vi "Webcam Management.vi"() -> ()   [LabVIEW 2014]
uses:
  <vilib>/vision/driver/IMAQdx.llb/IMAQdx Attribute Type.ctl
  <vilib>/userdefined/High Color/IMAQdx.ctl
  <vilib>/vision/driver/NI_Vision_Acquisition_Software.lvlib
  <resource>/objmgr/imaqdx.rc
panel:
  out "Brightness Mode":u32
  out "Contrast Mode":u32
  in  "Brightness":dbl
  in  "Contrast":dbl min=0.0 max=0.6 step=0.1
  out "Attribute Information Array":T2(array[cluster])
  out "Image":T3(plugin-control)
  in  "stop":bool
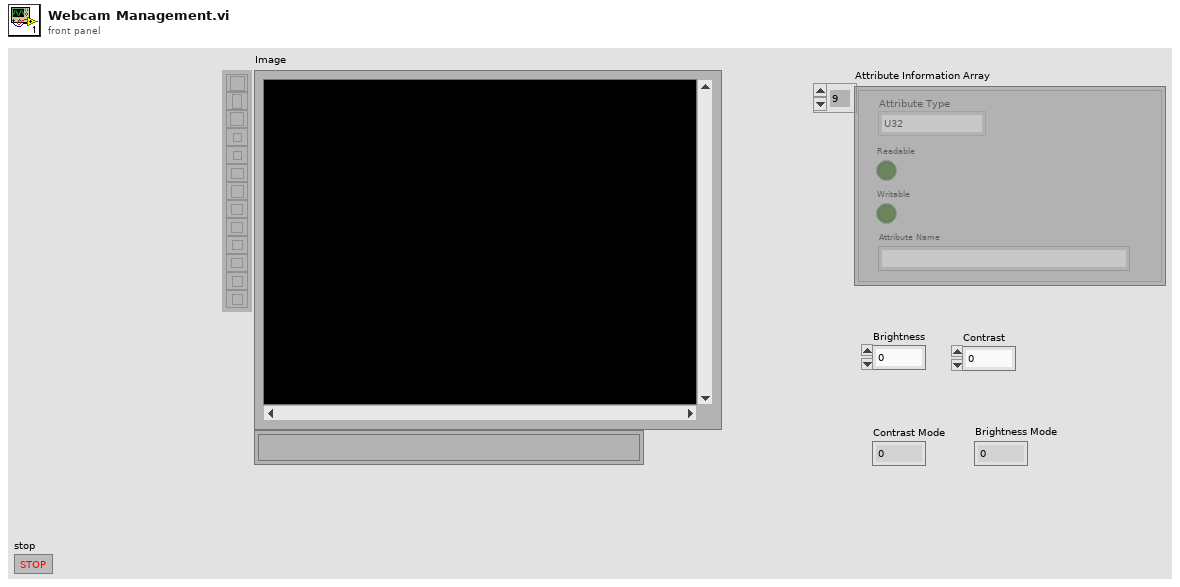
[diagram p1: front panel]
types:
  T1 = typedef "NI_Vision_Acquisition_Software.lvlib/IMAQdx Attribute Type.ctl" = enum32{"U32", "I64", "DBL", "String", "Enum", "Bool", "Command"}
  T2 = cluster{"Attribute Type":T1, "Readable":bool, "Writable":bool, "Attribute Name":string}[]
  T3 = typedef "IMAQ Image.ctl" = refnum<image>
  T4 = typedef "Image Type" = u32
  T5 = typedef "IMAQdx.ctl" = refnum<k21>
  T6 = cluster{"Global Rectangle":i32[], "Contours":cluster{"Contour Type":u32, "ROI Type":u32, "Points":i32[]}[]}
  T7 = cluster{"Global Rectangle[0]":i32, "Global Rectangle[1]":i32, "Global Rectangle[2]":i32, "Global Rectangle[3]":i32}
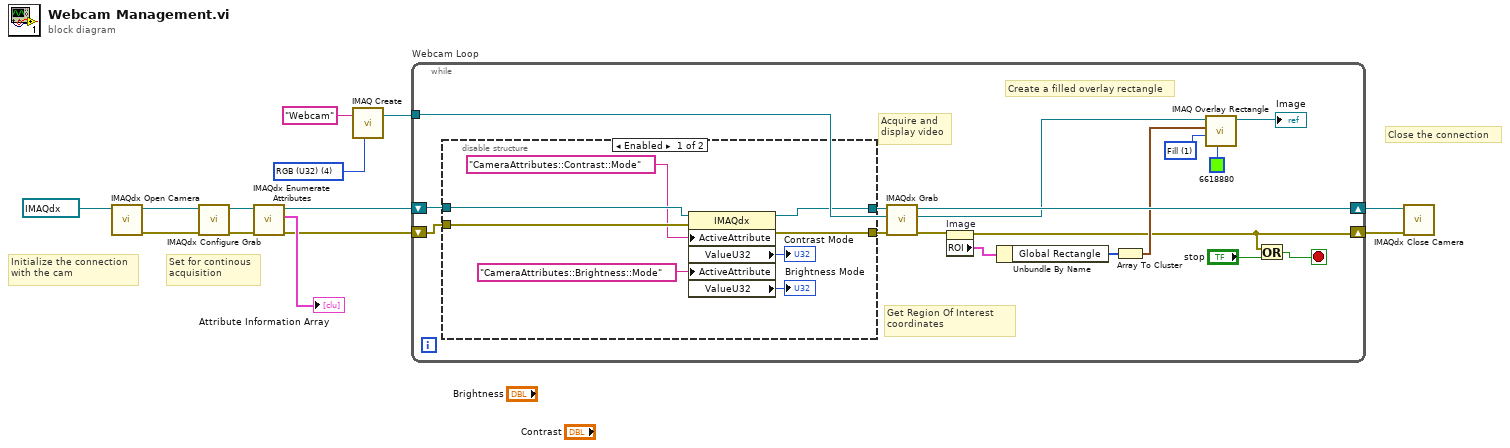
[diagram p0: block diagram]
diagram:
  w7 = T4 4 items=["Grayscale (U8)", "Grayscale (I16)", "Grayscale (SGL)", "Complex (CSG)", "RGB (U32)", "HSL (U32)", "RGB (U64)", "Grayscale (U16)"] ("Image Type")
  # "Close the connection"
  # "Set for continous\nacquisition"
  # "Initialize the connection\nwith the cam"
  n1 = call <vilib>:"IMAQdx Open Camera.vi"("Session In"=T5 "cam1") -> ("error out"=w12:errorcluster, "Session Out"=w13:T5)  [unwired: 9 in]
  n2 = call <vilib>:"IMAQdx Configure Grab.vi"("error in"=w12, "Session In"=w13) -> ("error out"=w5:errorcluster, "Session Out"=w4:T5)  [unwired: 8 in]
  n3 = call <vilib>:"IMAQdx Enumerate Attributes.vi"("error in"=w5, "Session In"=w4) -> ("error out"=w2:errorcluster, "Attribute Information Array"=→"Attribute Information Array":T2, "Session Out"=w1:T5)  [unwired: 7 in]
  n4 = call "IMAQ Create"("Image Name"="Webcam", "Image Type"=w7) -> ("New Image"=w8:T3)  [unwired: 3 in, 1 out]
  n5 = while "Webcam Loop" {
    shift-right: [w30] -> w10
    shift-left: w1 -> [w17]
    shift-right: [w18] -> w9
    shift-left: w2 -> [w14]
    tunnel: w8 -> [w29]
    stop <- w19 stop-if-true
    w22 = u32 1 items=["Frame", "Fill", "Highlight"] ("Drawing Mode (Frame)")
    # "Get Region Of Interest\ncoordinates"
    # "Create a filled overlay rectangle"
    # "Acquire and \ndisplay video"
    n6 = disable-structure shown="Enabled" {
      disable-tunnel: w17 -> [w38 w40]
      disable-tunnel: [w37 w40] -> w16
      disable-tunnel: [w36 w39] -> w15
      disable-tunnel: w14 -> [w35 w39]
      frame Enabled {
        n7 = property class="IMAQdx"(reference=w38, error in=w35, "ActiveAttribute"="CameraAttributes::Contrast::Mode", "ActiveAttribute"="CameraAttributes::Brightness::Mode") -> (reference out=w37:T5, error out=w36:errorcluster, "ValueU32"=→"Contrast Mode":u32, "ValueU32"=→"Brightness Mode":u32)
      }
      frame Disabled {
      }
    }
    n8 = call <vilib>:"IMAQdx Grab.vi"("error in"=w15, "Image In"=w29, "Session In"=w16) -> ("error out"=w28:errorcluster, "Image Out"=w23:T3, "Session Out"=w30:T5)  [unwired: 5 in, 1 out]
    n9 = property on="Image" class="ImageControl"(error in=w28) -> (error out=w18:errorcluster, "ROI"=w27:T6)  [unwired: 1 in, 1 out]
    n10 = Unbundle By Name(w27) -> ("Global Rectangle"=w26:i32[])
    n11 = Array To Cluster(array=w26) -> (cluster=w25:T7)
    n12 = call "IMAQ Overlay Rectangle"("Color"=u32 6618880, "Drawing Mode (Frame)"=w22, "Rectangle"=w25, "Image"=w23) -> ("Image Out"=→"Image":T3)  [unwired: 6 in, 1 out]
    n13 = Or(x=w18, y="stop") -> (x .or. y?=w19:bool)
  }
  n14 = call <vilib>:"IMAQdx Close Camera.vi"("error in"=w9, "Session In"=w10) -> ()  [unwired: 9 in, 1 out]
